vi "DIAdem Init Core.vi"(8 "error in":errorcluster) -> (0 "error out":errorcluster, 3 "DIAdem Reference":T1)   [LabVIEW 2011]
uses:
  <vilib>/ExportToExcel/DIAdem Reference.ctl
  Addons/DIAdem/DIAdem.llb/DIAdem String Variable Set.vi
  server lib/Spartan Version.vi
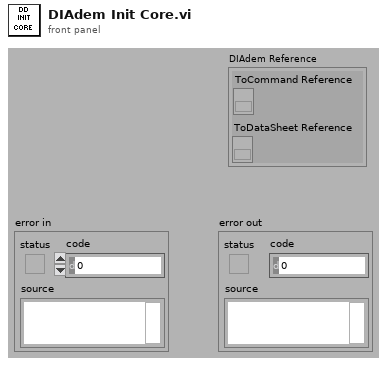
[diagram p1: front panel]
types:
  T1 = typedef "DIAdem Reference.ctl" = cluster{"ToCommand Reference":refnum<k7>, "ToDataSheet Reference":refnum<k7>}
  T2 = typedef "OGAB Version.ctl" = cluster{"Version":string, "Build Number":u32, "Build Date/Time":dbl}
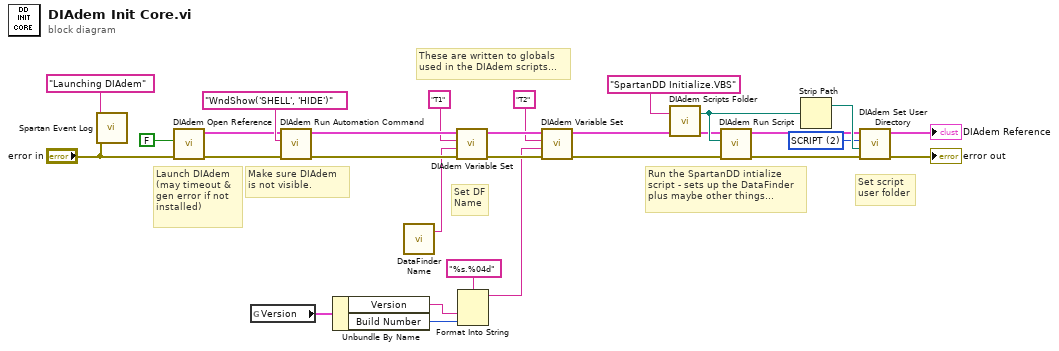
[diagram p0: block diagram]
diagram:
  w20 = u16 2 items=["NAVIGATOR", "REPORT", "SCRIPT"] ("DIAdem panel")
  # "These are written to globals\nused in the DIAdem scripts..."
  # "Set DF\nName"
  # "Run the SpartanDD intialize\nscript - sets up the DataFinder\nplus maybe other things..."
  # "Make sure DIAdem\nis not visible."
  # "Launch DIAdem\n(may timeout &\ngen error if not\ninstalled)"
  # "Set script\nuser folder"
  n1 = call "Spartan Event Log.vi"("error in (no error)"="error in", "message (\"\")"="Launching DIAdem" ("command")) -> ()  [unwired: 3 in, 4 out]
  n2 = call "DIAdem Open Reference.vi"("error in (no error)"="error in", "Show Environment (F)"=FALSE) -> ("error out"=w16:errorcluster, "DIAdem Reference"=w17:T1)  [unwired: 2 in, 6 out]
  n3 = global read "Spartan Version.vi" "Version"() -> (w5:T2)
  n4 = call "DIAdem Run Automation Command.vi"("error in (no error)"=w16, "command"="WndShow('SHELL', 'HIDE')", "DIAdem Reference"=w17) -> ("error out"=w24:errorcluster, "DIAdem Reference"=w23:T1)  [unwired: 7 out]
  n5 = Unbundle By Name(w5) -> ("Version"=w3:string, "Build Number"=w2:u32)
  n6 = call "DataFinder Name.vi"() -> ("DataFinder Name"=w11:string)  [unwired: 3 in]
  n7 = call-poly "DIAdem Variable Set.vi"("error in (no error)"=w24, "Value"=w11, "Variable Name"="T1", "DIAdem Reference"=w23) -> ("error out"=w10:errorcluster, "DIAdem Reference"=w8:T1)  [unwired: 6 out]
  n8 = Format Into String(format string="%s.%04d", w3, w2) -> (resulting string=w1:string)  [unwired: 2 in, 1 out]
  n9 = call-poly "DIAdem Variable Set.vi"("error in (no error)"=w10, "Value"=w1, "Variable Name"="T2", "DIAdem Reference"=w8) -> ("error out"=w9:errorcluster, "DIAdem Reference"=w7:T1)  [unwired: 6 out]
  n10 = call "DIAdem Scripts Folder.vi"("Relative Path (\"\" - Folder)"="SpartanDD Initialize.VBS" ("name or relative path")) -> ("Scripts Folder"=w27:path)  [unwired: 2 out]
  n11 = call "DIAdem Run Script.vi"("error in (no error)"=w9, "script file"=w27, "DIAdem Reference"=w7) -> ("error out"=w13:errorcluster, "DIAdem Reference"=w14:T1)  [unwired: 7 out]
  n12 = Strip Path(path=w27) -> (stripped path=w28:path)  [unwired: 1 out]
  n13 = call "DIAdem Set User Directory.vi"("error in (no error)"=w13, "user directory"=w28, "DIAdem panel"=w20, "DIAdem Reference"=w14) -> ("error out"=→"error out":errorcluster, "DIAdem Reference"=→"DIAdem Reference":T1)  [unwired: 6 out]
